vi "Actor Core.vi"(8 "error in":errorcluster, 11 "LEF HMI in":refnum<class "Supervision.lvclass">) -> (0 "error out":errorcluster, 3 "Actor out":refnum<class "Actor.lvclass">)   [LabVIEW 2020, in "Supervision.lvlib" / "Supervision.lvclass"]
uses:
  Supervision.lvclass
  D:/Projets/STEP AT/LUGE 2022.2/UIA_Demo/support/UI_Actor.lvlibp/UI_Actor/UI_Actor.lvclass
  D:/Projets/STEP AT/LUGE 2022.2/UIA_Demo/support/Actor Framework.lvlibp/1abvi3w/vi.lib/ActorFramework/Actor/Actor.lvclass
  support/Actor Framework.lvlibp/1abvi3w/vi.lib/ActorFramework/Actor/Actor.lvclass
  D&Cs/SCHEMA_01/SCHEMA_01/SCHEMA_01.lvclass
  support/UI_Actor.lvlibp/UI_Actor/UI_Actor.lvclass
  D&Cs/SCHEMA_02/SCHEMA_02/SCHEMA_02.lvclass
  D&Cs/SCHEMA_03/SCHEMA_03/SCHEMA_03.lvclass
  D&Cs/LiveDatActor/LiveDatActor/LiveDatActor.lvclass
  D&Cs/DualScreen/DualScreen/DualScreenParam.ctl
  D&Cs/SingleIndi/SingleIndi/SingleIndi.lvclass
  D&Cs/DualScreenH/DualScreenH/DualScreenH.lvclass
  support/Graph Actor.lvlibp/Graph Actor/Children/GRT2/GRT2/GRT2.lvclass
  support/UI_Actor.lvlibp/UI_Actor/Read AppPath.vi
  support/UI_Actor.lvlibp/UI_Actor/Read UE Ref.vi
  support/UI_Actor.lvlibp/UI_Actor Messages/UI_Resize Msg/UI_Resize Msg.lvclass
  support/Actor Framework.lvlibp/1abvi3w/vi.lib/ActorFramework/Stop Msg/Stop Msg.lvclass
  support/UI_Actor.lvlibp/UI_Actor Messages/UI_ShowIn_Subpanel Msg/UI_ShowIn_Subpanel Msg.lvclass
  D:/Projets/STEP AT/LUGE 2022.2/UIA_Demo/Supervision/Supervision/Supervision.lvclass
  support/Graph Actor.lvlibp/Graph Actor/Tools/GRT2_BuffMan/GRT2_BuffMan/GRT2_BuffMan.lvclass
  D&Cs/DualScreen/DualScreen/DualScreen.lvclass
panel:
  in  "D&C list":i32(listbox)
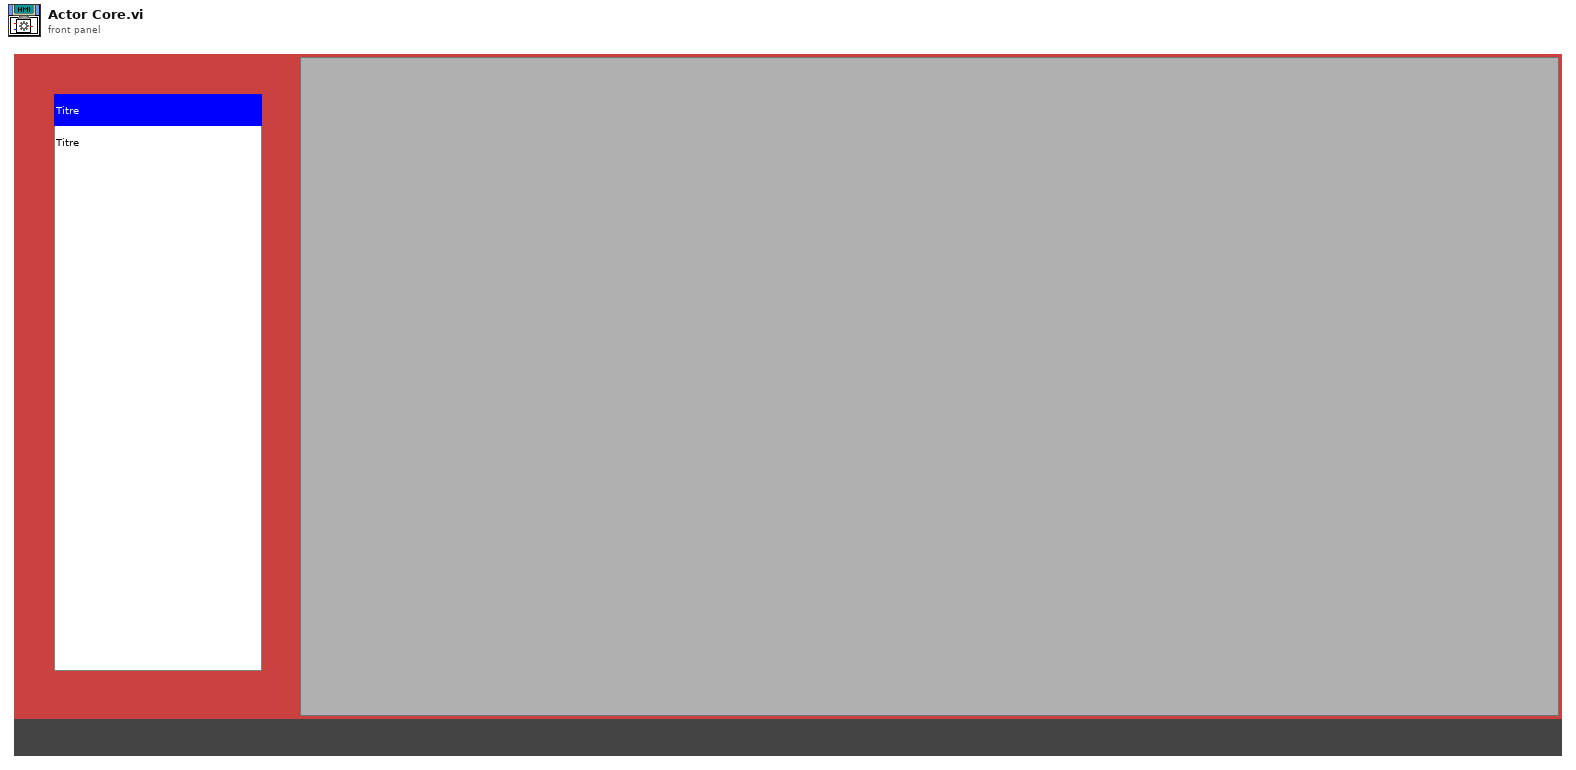
[diagram p1: front panel]
types:
  T1 = cluster{"Panes sizing":enum16{"Sticks Top/Left", "Sticks Bottom/Right", "Proportional"}, "Splitter Position":i32, "Splitter Locked":bool}
  T2 = typedef "DualScreen.lvlib/DualScreen.lvclass/DualScreenParam.ctl" = cluster{"1st UIA":refnum<class "UI_Actor.lvclass">, "2nd UIA":refnum<class "UI_Actor.lvclass">, "Splitter params":cluster{"Panes sizing":enum16{"Sticks Top/Left", "Sticks Bottom/Right", "Proportional"}, "Splitter Position":i32, "Splitter Locked":bool}}
  T3 = cluster{"Dual Screen out":refnum<class "UI_Actor.lvclass">, string}
  T4 = cluster{"Dual Screen out":refnum<class "UI_Actor.lvclass">, string}[]
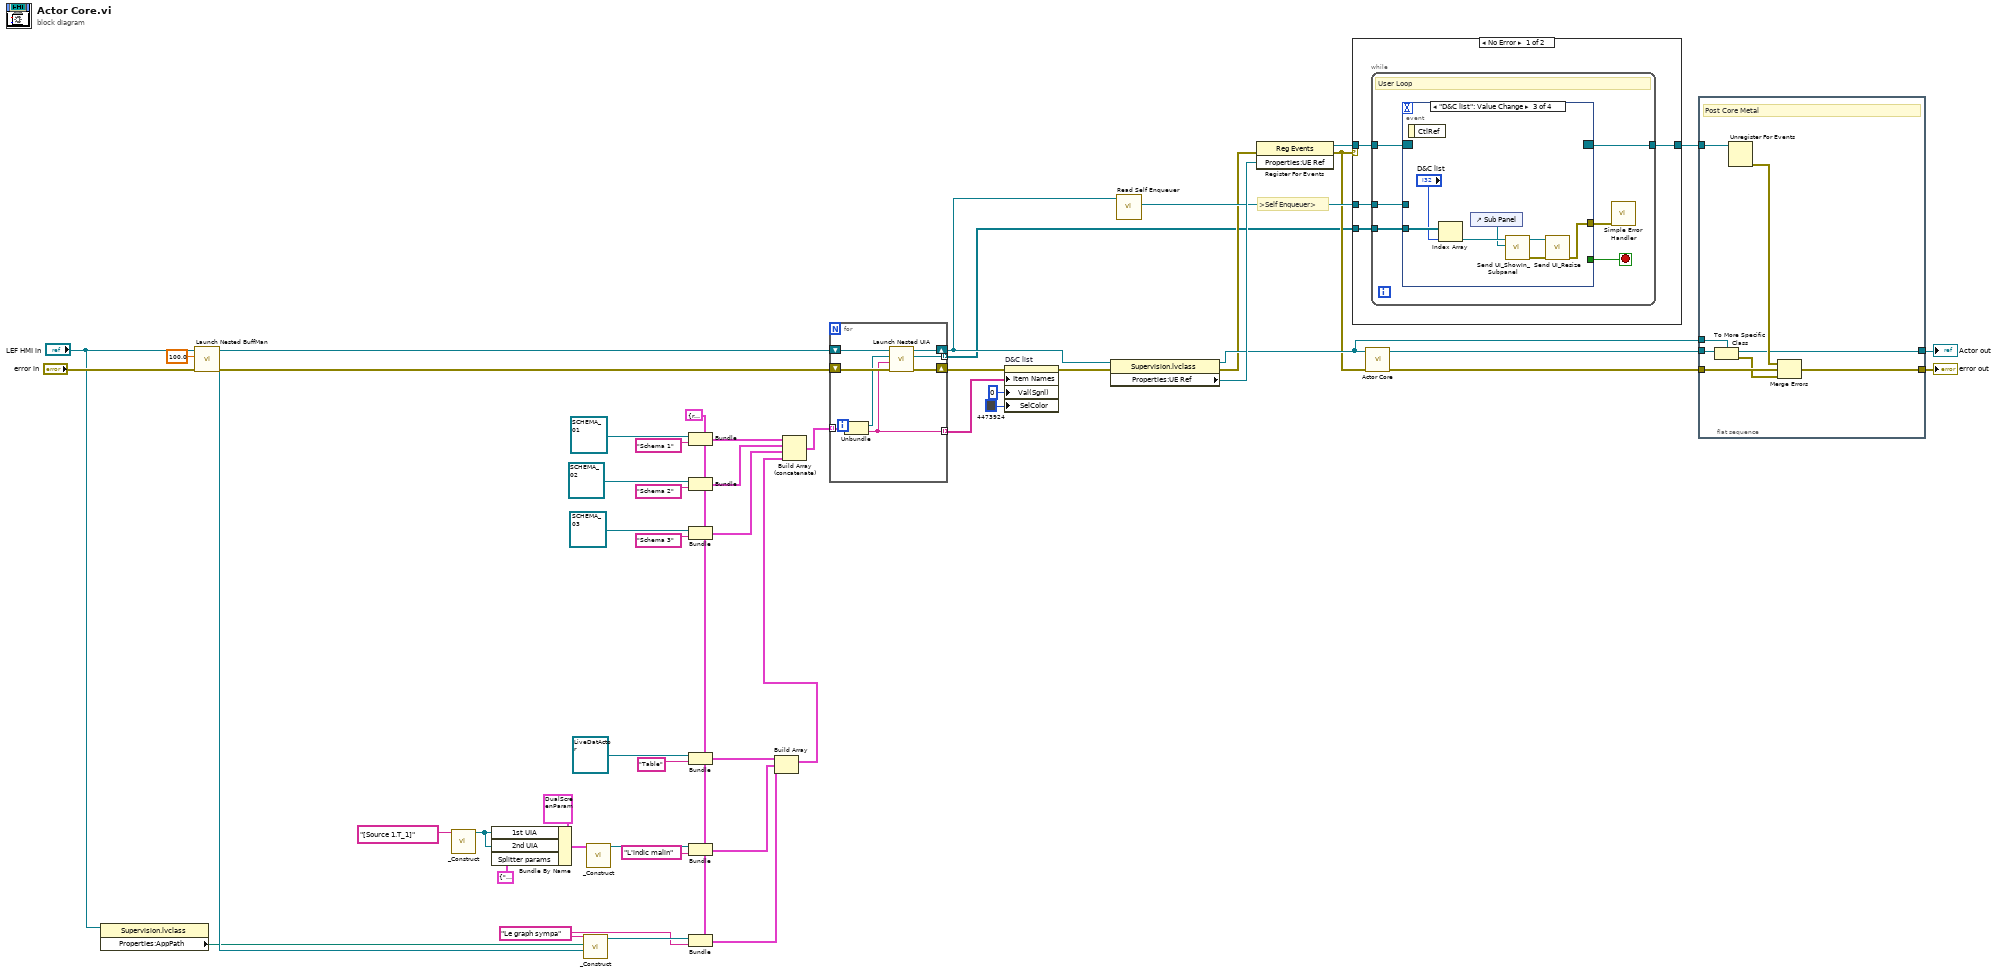
[diagram p0: block diagram]
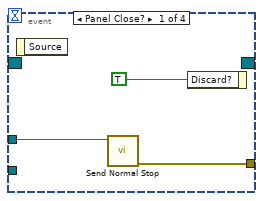
[diagram p2: hidden frame]
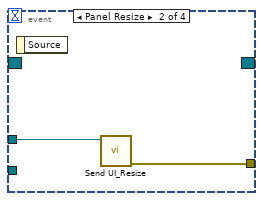
[diagram p3: hidden frame]
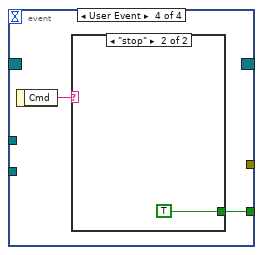
[diagram p4: hidden frame]
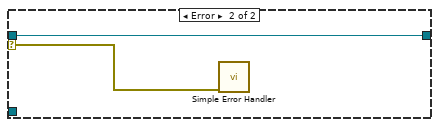
[diagram p6: hidden frame]
diagram:
  w13 = "Le graph sympa"
  w14 = T3 {"Dual Screen out"=refnum, ""}
  # ">Self Enqueuer>"
  n1 = property class="Supervision.lvclass"(reference="LEF HMI in") -> ("Properties:AppPath"=w10:path)  [unwired: 1 in, 2 out]
  n2 = call "Launch Nested BuffMan.vi"("error in (no error)"="error in", "Depth (s)"=100.0, "Caller In"="LEF HMI in") -> ("error out"=w17:errorcluster, "Thesaurus"=w16:refnum<class "ThesaurusDB.lvclass">, "Caller Out"=w19:refnum<class "Supervision.lvclass">)  [unwired: 6 in]
  n3 = call "_Construct.vi"("ChanSel init"="[Source 1.T_1]") -> ("SingleIndi out"=w9:refnum<class "SingleIndi.lvclass">)  [unwired: 9 in, 1 out]
  n4 = Bundle By Name(cluster=T2 {"1st UIA"=refnum, "2nd UIA"=refnum, "Splitter params"={"Panes sizing"=enum."Sticks Top/Left", "Splitter Position"=0, "Splitter Locked"=FALSE}} ("Parameters"), "1st UIA"=w9, "2nd UIA"=w9, "Splitter params"=T1 {"Panes sizing"=enum."Sticks Top/Left", "Splitter Position"=340, "Splitter Locked"=FALSE}) -> (w8:T2)
  n5 = call "_Construct.vi"("Thesaurus"=w16, "Save folder"=w10, "Name"=w13) -> ("GRT2 out"=w15:refnum<class "GRT2.lvclass">)  [unwired: 7 in, 1 out]
  n6 = call "_Construct.vi"("Parameters"=w8) -> ("Dual Screen out"=w5:refnum<class "DualScreenH.lvclass">)  [unwired: 9 in, 1 out]
  n7 = Bundle(cluster=w14, "Dual Screen out"=refnum<class "SCHEMA_01.lvclass"> refnum ("SCHEMA_01.lvlib:SCHEMA_01.lvclass"), "Schema 1") -> (w36:T3)
  n8 = Bundle(cluster=w14, "Dual Screen out"=refnum<class "SCHEMA_02.lvclass"> refnum ("SCHEMA_02.lvlib:SCHEMA_02.lvclass"), "Schema 2") -> (w30:T3)
  n9 = Bundle(cluster=w14, "Dual Screen out"=refnum<class "SCHEMA_03.lvclass"> refnum ("SCHEMA_03.lvlib:SCHEMA_03.lvclass"), "Schema 3") -> (w31:T3)
  n10 = Bundle(cluster=w14, "Dual Screen out"=refnum<class "LiveDatActor.lvclass"> refnum ("LiveDatActor.lvlib:LiveDatActor.lvclass"), "Table") -> (w4:T3)
  n11 = Bundle(cluster=w14, "Dual Screen out"=w5, "L'indic malin") -> (w3:T3)
  n12 = Bundle(cluster=w14, "Dual Screen out"=w15, w13) -> (w2:T3)
  n13 = Build Array(w4, w3, w2) -> (w1:T4)
  n14 = Build Array (concatenate)(w36, w30, w31, w1) -> (w35:T4)
  n15 = for {
    shift-right: [w59] -> w38
    shift-left: w19 -> [w58]
    shift-right: [w56] -> w24
    shift-left: w17 -> [w57]
    tunnel: w35 -> [w53] mode=indexing
    tunnel: [w52] -> w25 mode=indexing
    tunnel: [w55] -> w22 mode=indexing
    n16 = Unbundle(w53) -> ("Dual Screen out"=w54:refnum<class "UI_Actor.lvclass">, w52:string)
    n17 = call "Launch Nested UIA.vi"("error in (no error)"=w57, "Name"=w52, "UI_Actor"=w54, "Caller UIA in"=w58) -> ("error out"=w56:errorcluster, "Nested Actor's Enqueuer"=w55:refnum<class "Message Enqueuer.lvclass">, "Caller UIA out"=w59:refnum<class "Supervision.lvclass">)  [unwired: 5 in]
  }
  n18 = property on="D&C list" class="LstBox (strict)"(error in=w24, "Item Names"=w25, "Val(Sgnl)"=0 ("Value (Signaling)"), "SelColor"=u32 4473924 ("Selection Color")) -> (error out=w39:errorcluster)  [unwired: 1 in, 1 out]
  n19 = property on="Property Node" class="Supervision.lvclass"(reference=w38, error in=w39) -> (reference out=w44:refnum<class "Supervision.lvclass">, error out=w41:errorcluster, "Properties:UE Ref"=w45:refnum<user-event>)
  n20 = call "Read Self Enqueuer.vi"("Actor"=w38) -> ("Self Enqueuer"=w43:refnum<class "Message Enqueuer.lvclass">)  [unwired: 10 in]
  n21 = register-events(error in=w41, w45) -> (reference out=w50:refnum<event-registration>, error out=w42:errorcluster)  [unwired: 1 in]
  n22 = case shown="No Error" w42 {
    selector: w42 -> [_ w85]
    tunnel: w50 -> [w63 w86]
    tunnel: [w62 w86] -> w51
    tunnel: w43 -> [w61 _]
    tunnel: w22 -> [w60 _]
    frame No Error {
      n23 = while {
        tunnel: w61 -> [w68]
        tunnel: w63 -> [w66]
        tunnel: [w65] -> w62
        tunnel: w60 -> [w64]
        stop <- w69 stop-if-true
        # "User Loop"
        n24 = event shown="[2] \"D&C list\": Value Change" {
          selector: w66 -> [_ _ _ _]
          dyn-events: [_ _ _ _] -> w65
          timeout: _ -> [_ _ _ _]
          tunnel: [_ _ _ w82] -> w69
          tunnel: w68 -> [w71 w74 _ _]
          tunnel: [w70 w73 w76 _] -> w67
          tunnel: w64 -> [_ _ w79 _]
          event Panel Close? {
            n25 = event-data() -> ()  [unwired: 1 in, 1 out]
            n26 = call "Send Normal Stop.vi"("Message Enqueuer"=w71) -> ("error out"=w70:errorcluster)  [unwired: 10 in]
            n27 = event-data("Discard?"=TRUE) -> ()  [unwired: 1 in, 1 out]
          }
          event Panel Resize {
            n28 = event-data() -> ()  [unwired: 1 in, 1 out]
            n29 = call "Send UI_Resize.vi"("Message Enqueuer"=w74) -> ("error out"=w73:errorcluster)  [unwired: 9 in, 1 out]
          }
          event "D&C list": Value Change {
            n30 = event-data() -> ()  [unwired: 1 in, 1 out]
            n31 = Index Array(array=w79, index="D&C list") -> (element=w77:refnum<class "Message Enqueuer.lvclass">)
            n32 = control-ref of="Sub Panel"() -> (w75:refnum<vi>)
            n33 = call "Send UI_ShowIn_Subpanel.vi"("Sub Panel"=w75, "Message Enqueuer"=w77) -> ("error out"=w81:errorcluster, "Message Enqueuer out"=w80:refnum<class "Message Enqueuer.lvclass">)  [unwired: 8 in]
            n34 = call "Send UI_Resize.vi"("error in (no error)"=w81, "Message Enqueuer"=w80) -> ("error out"=w76:errorcluster)  [unwired: 8 in, 1 out]
          }
          event User Event {
            n35 = event-data() -> ("Cmd"=w83:string)  [unwired: 1 in]
            n36 = case shown="\"stop\"" w83 {
              tunnel: [_ TRUE] -> w82
              frame Default {
              }
              frame "stop" {
              }
            }
          }
        }
        n37 = call <vilib>:"Simple Error Handler.vi"("error in (no error)"=w67) -> ()  [unwired: 4 in, 5 out]
      }
    }
    frame Error {
      n38 = call <vilib>:"Simple Error Handler.vi"("error in (no error)"=w85) -> ()  [unwired: 4 in, 5 out]
    }
  }
  n39 = call-parent "Actor Core.vi"("error in"=w42, "UI_Actor in"=w44) -> ("error out"=w49:errorcluster, "Actor out"=w48:refnum<class "Actor.lvclass">)  [unwired: 8 in]
  n40 = flat-sequence {
    tunnel: [w87] -> w47
    tunnel: w48 -> [w94]
    tunnel: w49 -> [w92]
    tunnel: w44 -> [w93]
    tunnel: [w90] -> w46
    tunnel: w51 -> [w89]
    frame #0 {
      # "Post Core Metal"
      n41 = To More Specific Class(target class=w93, reference=w94) -> (specific class reference=w87:refnum<class "Supervision.lvclass">, error out=w91:errorcluster)  [unwired: 1 in]
      n42 = Unregister For Events(event registration refnum=w89) -> (error out=w88:errorcluster)  [unwired: 1 in]
      n43 = Merge Errors(w88, w92, w91) -> (w90:errorcluster)
    }
  }
  "error out" <- w46
  "Actor out" <- w47
